vi "Generate Board.vi"(7 "Board Array":i16[][](array[numeric]), 11 "Piece Array":i16[][](array[numeric])) -> (3 "Picture":picture)   [LabVIEW 2019]
panel:
  in  "Block Size":u32=20
  in  "Color Array":u32[](array[colorbox])=[0, 15790080, 8388608, 8421376, 128, 32896, 8388736, 32896]
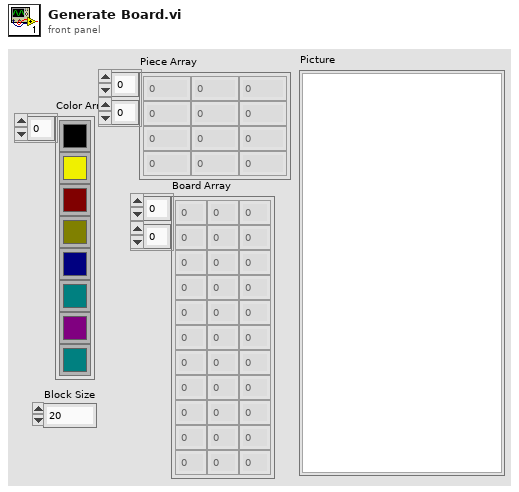
[diagram p1: front panel]
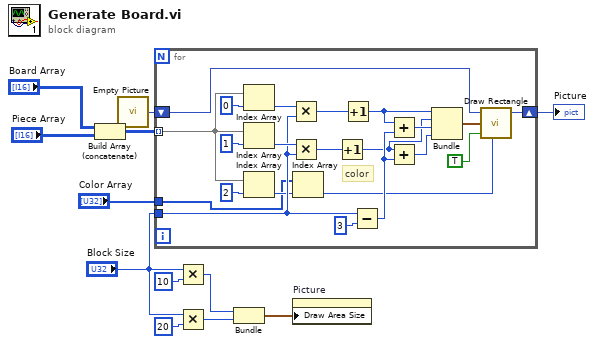
[diagram p0: block diagram]
diagram:
  n1 = Build Array (concatenate)("Board Array", "Piece Array") -> (w4:i16[][])
  n2 = call "Empty Picture"() -> ("empty picture"=w11:picture)
  n3 = for {
    shift-right: [w13] -> w12
    shift-left: w11 -> [w15]
    tunnel: w4 -> [w31] mode=indexing
    tunnel: "Block Size" -> [w24]
    tunnel: "Color Array" -> [w16]
    # "color"
    n4 = Index Array(array=w31, index=0) -> (element=w28:i16)
    n5 = Index Array(array=w31, index=1) -> (element=w27:i16)
    n6 = Index Array(array=w31, index=2) -> (element=w17:i16)
    n7 = Multiply(x=w28, y=w24) -> (x*y=w25:u32)
    n8 = Multiply(x=w27, y=w24) -> (x*y=w26:u32)
    n9 = Index Array(array=w16, index=w17) -> (element=w14:u32)
    n10 = Increment(x=w26) -> (x+1=w20:u32)
    n11 = Increment(x=w25) -> (x+1=w21:u32)
    n12 = Subtract(x=w24, y=u32 3) -> (x-y=w29:u32)
    n13 = Add(x=w21, y=w29) -> (x+y=w22:u32)
    n14 = Add(x=w20, y=w29) -> (x+y=w23:u32)
    n15 = Bundle(w21, w20, w22, w23) -> (w19:cluster{u32, u32, u32, u32})  [unwired: 1 in]
    n16 = call <vilib>:"Draw Rectangle.vi"("picture"=w15, "rect"=w19, "fill?(F)"=TRUE, "color(black)"=w14) -> ("new picture"=w13:picture)  [unwired: 5 in]
  }
  "Picture" <- w12
  n17 = Multiply(x="Block Size", y=u32 10) -> (x*y=w9:u32)
  n18 = Multiply(x="Block Size", y=u32 20) -> (x*y=w10:u32)
  n19 = Bundle(w9, w10) -> (w6:cluster{u32, u32})  [unwired: 1 in]
  n20 = property on="Picture" class="Pict"("Draw Area Size"=w6) -> ()  [unwired: 2 in, 2 out]
